vi "Execute.vi"(8 "Active?":bool, 9 "cfs":dbl[](array[numeric]), 10 "Inputs":dbl[](array[numeric]), 11 "Cerebellum in":refnum<class "Cerebellum.lvclass">) -> (1 "PC Left":dbl, 2 "PC Right":dbl, 3 "Cerebellum out":refnum<class "Cerebellum.lvclass">)   [LabVIEW 2013, in "Cerebellum.lvclass"]
uses:
  Cerebellum.lvclass
  Cerebellum.lvclass/Cerebellum.ctl
  AER/AER.lvclass
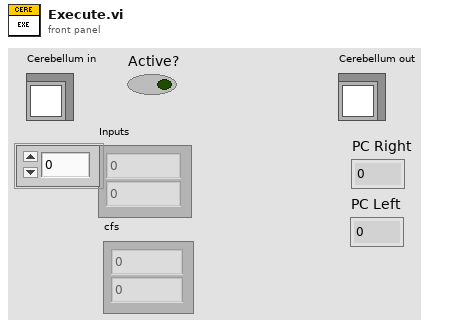
[diagram p1: front panel]
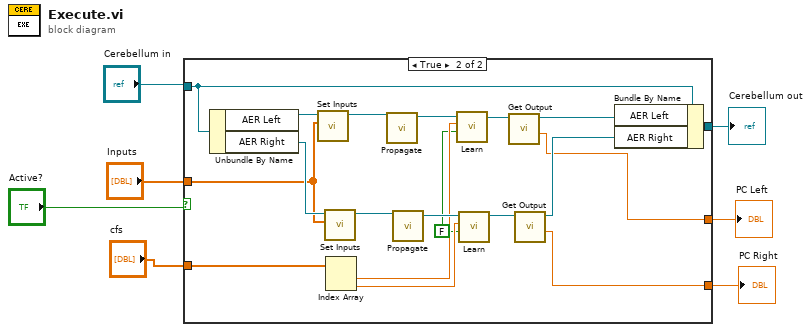
[diagram p0: block diagram]
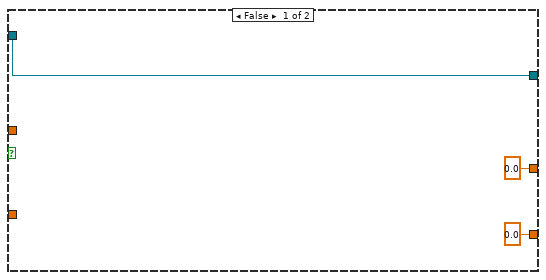
[diagram p2: hidden frame]
diagram:
  n1 = case shown="True" "Active?" {
    tunnel: "Cerebellum in" -> [w10 w29]
    tunnel: [w10 w27] -> w6
    tunnel: "Inputs" -> [_ w23]
    tunnel: [0.0 ("AvePC") w18] -> w4
    tunnel: [0.0 ("AvePC") w17] -> w3
    tunnel: "cfs" -> [_ w16]
    frame False {
    }
    frame True {
      w11 = FALSE ("Learning?")
      n2 = Unbundle By Name(w29) -> ("AER Left"=w28:refnum<class "AER.lvclass">, "AER Right"=w25:refnum<class "AER.lvclass">)
      n3 = call "Set Inputs.vi"("Inputs"=w23, "AER in"=w28) -> ("AER out"=w26:refnum<class "AER.lvclass">)  [unwired: 9 in]
      n4 = call "Set Inputs.vi"("Inputs"=w23, "AER in"=w25) -> ("AER out"=w24:refnum<class "AER.lvclass">)  [unwired: 9 in]
      n5 = Index Array(array=w16) -> (element #1=w15:dbl, element #2=w14:dbl)  [unwired: 2 in]
      n6 = call "Propagate.vi"("AER in"=w26) -> ("AER out"=w22:refnum<class "AER.lvclass">)  [unwired: 10 in]
      n7 = call "Propagate.vi"("AER in"=w24) -> ("AER out"=w21:refnum<class "AER.lvclass">)  [unwired: 10 in]
      n8 = call "Learn.vi"("Learning?"=w11, "cf"=w15, "AER in"=w22) -> ("AER out"=w13:refnum<class "AER.lvclass">)  [unwired: 8 in]
      n9 = call "Learn.vi"("Learning?"=w11, "cf"=w14, "AER in"=w21) -> ("AER out"=w12:refnum<class "AER.lvclass">)  [unwired: 8 in]
      n10 = call "Get Output.vi"("AER in"=w13) -> ("AvePC"=w18:dbl, "AER out"=w20:refnum<class "AER.lvclass">)  [unwired: 8 in, 1 out]
      n11 = call "Get Output.vi"("AER in"=w12) -> ("AvePC"=w17:dbl, "AER out"=w19:refnum<class "AER.lvclass">)  [unwired: 8 in, 1 out]
      n12 = Bundle By Name(cluster=w29, "AER Left"=w20, "AER Right"=w19) -> (w27:refnum<class "Cerebellum.lvclass">)
    }
  }
  "Cerebellum out" <- w6
  "PC Left" <- w4
  "PC Right" <- w3
